vi "Levelmeter_Merge_Cluster.vi"(1 "Mischer Levelmeter  Control":T2={"N-Shield Refill"=FALSE, "Automatic Refill Shield"=TRUE, "Trap Refill"=FALSE, "Automatic Refill Trap"=TRUE}, 2 "Mischer Levelmeter Status":T1) -> (0 "Mischer Levelmeter":T3={"Plot"=[], "N-Shield (%)"=0.0, "He (%)"=0.0, "Coldtrap (%)"=0.0, "He - POT (%)"=0.0, "N-Shield Refill"=FALSE, "Last fill Shield"="", "Auto Refill Shield"=TRUE, "Trap Refill"=FALSE, "Last fill Coldtrap"="", "Auto Refill Trap"=TRUE, "Shield Refill"=FALSE, "Coldtrap Refill"=FALSE, "Auto Trap activatet"=FALSE, "Auto Shield Activatet"=FALSE})   [LabVIEW 2019]
uses:
  Mischer/Mischer_Levelmeter-Cluster.ctl
  Mischer/Mischer_Levelmeter_Control.ctl
  Mischer/Mischer_Levelmeter_Status.ctl
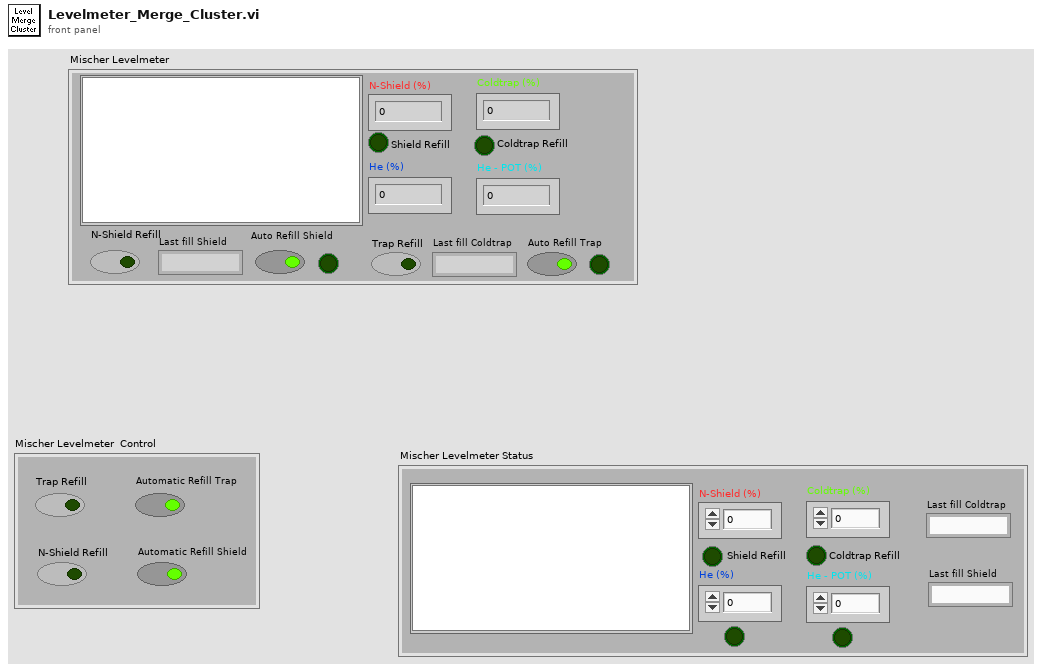
[diagram p1: front panel]
types:
  T1 = typedef "Mischer_Levelmeter_Status.ctl" = cluster{"Plot":dbl[][], "N-Shield (%)":dbl, "He (%)":dbl, "Coldtrap (%)":dbl, "He - POT (%)":dbl, "Shield Refill":bool, "Coldtrap Refill":bool, "Last fill Shield":string, "Last fill Coldtrap":string, "Auto Shield refill Activatet":bool, "Auto Trap refill activatet":bool}
  T2 = typedef "Mischer_Levelmeter_Control.ctl" = cluster{"N-Shield Refill":bool, "Automatic Refill Shield":bool, "Trap Refill":bool, "Automatic Refill Trap":bool}
  T3 = typedef "Mischer_Levelmeter-Cluster.ctl" = cluster{"Plot":dbl[][], "N-Shield (%)":dbl, "He (%)":dbl, "Coldtrap (%)":dbl, "He - POT (%)":dbl, "N-Shield Refill":bool, "Last fill Shield":string, "Auto Refill Shield":bool, "Trap Refill":bool, "Last fill Coldtrap":string, "Auto Refill Trap":bool, "Shield Refill":bool, "Coldtrap Refill":bool, "Auto Trap activatet":bool, "Auto Shield Activatet":bool}
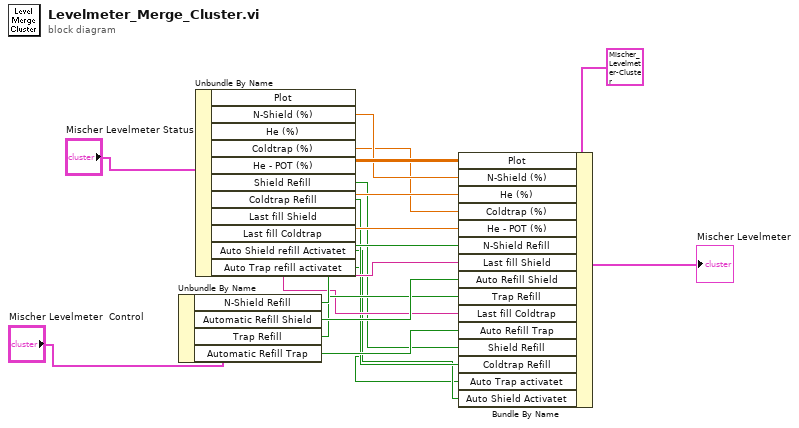
[diagram p0: block diagram]
diagram:
  n1 = Unbundle By Name("Mischer Levelmeter  Control") -> ("N-Shield Refill"=w10:bool, "Automatic Refill Shield"=w9:bool, "Trap Refill"=w8:bool, "Automatic Refill Trap"=w7:bool)
  n2 = Unbundle By Name("Mischer Levelmeter Status") -> ("Plot"=w15:dbl[][], "N-Shield (%)"=w14:dbl, "He (%)"=w13:dbl, "Coldtrap (%)"=w12:dbl, "He - POT (%)"=w11:dbl, "Shield Refill"=w4:bool, "Coldtrap Refill"=w3:bool, "Last fill Shield"=w6:string, "Last fill Coldtrap"=w5:string, "Auto Shield refill Activatet"=w2:bool, "Auto Trap refill activatet"=w1:bool)
  n3 = Bundle By Name(cluster=T3 {"Plot"=array4x34874[139496 elements], "N-Shield (%)"=0.0, "He (%)"=99.97689819335938, "Coldtrap (%)"=0.0, "He - POT (%)"=98.66000366210938, "N-Shield Refill"=FALSE, "Last fill Shield"="", "Auto Refill Shield"=TRUE, "Trap Refill"=FALSE, "Last fill Coldtrap"="", "Auto Refill Trap"=TRUE, "Shield Refill"=FALSE, "Coldtrap Refill"=FALSE, "Auto Trap activatet"=FALSE, "Auto Shield Activatet"=FALSE} ("Mischer Levelmeter 2"), "Plot"=w15, "N-Shield (%)"=w14, "He (%)"=w13, "Coldtrap (%)"=w12, "He - POT (%)"=w11, "N-Shield Refill"=w10, "Last fill Shield"=w6, "Auto Refill Shield"=w9, "Trap Refill"=w8, "Last fill Coldtrap"=w5, "Auto Refill Trap"=w7, "Shield Refill"=w4, "Coldtrap Refill"=w3, "Auto Trap activatet"=w1, "Auto Shield Activatet"=w2) -> (→"Mischer Levelmeter":T3)
